vi "id2coor.vi"(2 "Id":i32=1, 3 "Size (x,y,z)":dbl[](array[numeric])=[100.0, 100.0, 100.0]) -> (0 "Position (x,y,z)":i32[](array[numeric])=[1, 0, 0])   [LabVIEW 2013]
doc: "Get the position (x,y,z) corresponding to the input Id"
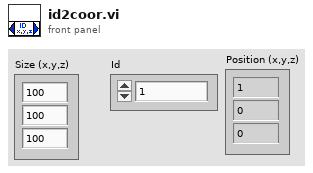
[diagram p1: front panel]
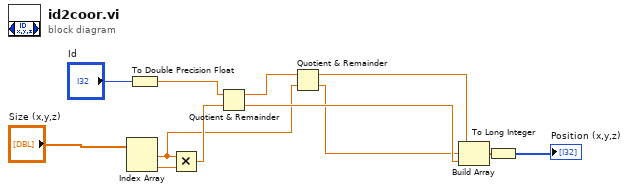
[diagram p0: block diagram]
diagram:
  n1 = Index Array(array="Size (x,y,z)") -> (element #1=w6:dbl, element #2=w10:dbl)  [unwired: 2 in]
  n2 = To Double Precision Float(number="Id") -> (double precision float=w1:dbl)
  n3 = Multiply(x=w6, y=w10) -> (x*y=w9:dbl)
  n4 = Quotient & Remainder(x=w1, y=w9) -> (x-y*floor(x/y)=w7:dbl, floor(x/y)=w8:dbl)
  n5 = Quotient & Remainder(x=w7, y=w6) -> (x-y*floor(x/y)=w4:dbl, floor(x/y)=w5:dbl)
  n6 = Build Array(w4, w5, w8) -> (w3:dbl[])
  n7 = To Long Integer(number=w3) -> (32bit integer=→"Position (x,y,z)":i32[])
